vi "Test 2.vi"() -> ()   [LabVIEW 2013, in "Generic Data Logger.lvlib" / "Generic Data Logger.lvclass"]
uses:
  Generic Data Logger.lvclass
  <instrlib>/Fluke 2625A/Fluke 2625A.lvlib
  Generic Instrument/Generic Instrument.lvclass
panel:
  in  "write buffer":string
  out "error out":errorcluster
  out "read buffer":string
  in  "VISA resource name":refnum<visa-resource-name>
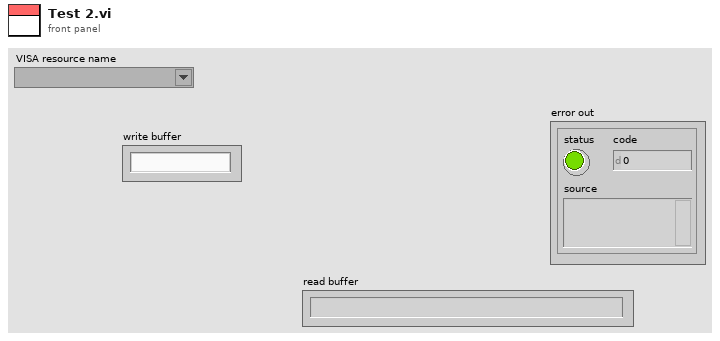
[diagram p1: front panel]
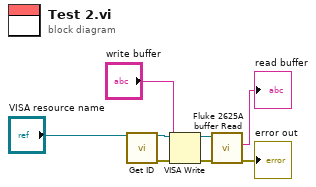
[diagram p0: block diagram]
diagram:
  n1 = call "Get ID.vi"("VISA resource name"="VISA resource name") -> ("VISA resource name 2"=w3:refnum<visa-resource-name>, "error out"=w2:errorcluster)  [unwired: 10 in, 3 out]
  n2 = VISA Write(VISA resource name=w3, write buffer="write buffer", error in (no error)=w2) -> (VISA resource name out=w7:refnum<visa-resource-name>, error out=w6:errorcluster)  [unwired: 1 out]
  n3 = call <instrlib>:"Fluke 2625A buffer Read.vi"("error out"=w6, "VISA resource name out"=w7) -> ("error out 2"=→"error out":errorcluster, "read buffer"=→"read buffer":string)  [unwired: 7 in, 1 out]
